vi "sub_imu_data-check.vi"(11 "str":string) -> (3 "val":bool)   [LabVIEW 2019]
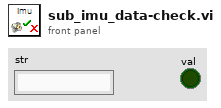
[diagram p1: front panel]
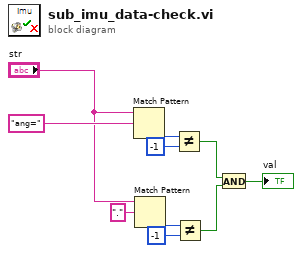
[diagram p0: block diagram]
diagram:
  n1 = Match Pattern(string="str", regular expression="ang=" ("정규식")) -> (offset past match=w9:i32)  [unwired: 1 in, 3 out]
  n2 = Match Pattern(string="str", regular expression="." ("정규식")) -> (offset past match=w6:i32)  [unwired: 1 in, 3 out]
  n3 = Not Equal?(x=w9, y=-1) -> (x != y?=w2:bool)
  n4 = Not Equal?(x=w6, y=-1) -> (x != y?=w3:bool)
  n5 = And(x=w2, y=w3) -> (x .and. y?=→"val":bool)
